vi "copy-data-eventSD.vi"(1 "cluster in":T1={"Kinetics"=[], "Spectrum"=[], "Experiments groups"=[], "GRAPH EXPERIMENTAL DATA"=[], "error out"={"status"=FALSE, "code"=0, "source"=""}, "group"=0, "exp selected"=0, "# exp"=0, "kinetics plot names"=[], "spectra plot names"=[], "FromToWave"={"FromWave"=0.0, "ToWave"=0.0}, "Laser shutter task"="", "Accelerator task"="", "Motor task"="", "GRAPH EXPERIMENTAL DATA ref"=refnum, "timedelays"=[0.0, 0.0, 0.0, 0.0, 0.0, 0.0, 0.0, 0.06019061100911815, 0.0521779104562645, 0.045231877429679615, 0.03921051490799832, 0.033990728811568754, 0.029465811603150715, 0.025543260876973825, 0.02214288834180205, 0.01919518054014414, 0.016639877791965713, 0.014424742312398925, 0.012504490320209958, 0.010839866306230088, 0.009396840537117498, 0.008145913389103785, 0.00706151229029317, 0.006121468943269439, 0.005306566140927374, 0.004600144911132549, 0.003987763959109073, 0.0034569044455719407, 0.00299671406541447, 0.0025977851951783253, 0.0022519625739982996, 0.00195217658646366, 0.0016922987392150965, 0.0014670163768006634, 0.0012717240756200802, 0.0011024294957352762, 0.0009556717658856477, 0.0008284507332614981, 0.0007181656316962257, 0.0006225619144775864, 0.0005396851648867825, 0.00046784114226338394, 0.0004055611468220084, 0.0003515719951773376, 0.00030476999279031153, 0.00026419837125694315, 0.00022902772919263772, 0.0001985390768670671, 0.0001721091379728629, 0.00014919760805372974, 0.00012933610911736794], "wavelengths"=[0.0, 0.0, 0.0, 0.0, 0.0, 0.0, 0.0, 0.06019061100911815, 0.0521779104562645, 0.045231877429679615, 0.03921051490799832, 0.033990728811568754, 0.029465811603150715, 0.025543260876973825, 0.02214288834180205, 0.01919518054014414, 0.016639877791965713, 0.014424742312398925, 0.012504490320209958, 0.010839866306230088, 0.009396840537117498, 0.008145913389103785, 0.00706151229029317, 0.006121468943269439, 0.005306566140927374, 0.004600144911132549, 0.003987763959109073, 0.0034569044455719407, 0.00299671406541447, 0.0025977851951783253, 0.0022519625739982996, 0.00195217658646366, 0.0016922987392150965, 0.0014670163768006634, 0.0012717240756200802, 0.0011024294957352762, 0.0009556717658856477, 0.0008284507332614981, 0.0007181656316962257, 0.0006225619144775864, 0.0005396851648867825, 0.00046784114226338394, 0.0004055611468220084, 0.0003515719951773376, 0.00030476999279031153, 0.00026419837125694315, 0.00022902772919263772, 0.0001985390768670671, 0.0001721091379728629, 0.00014919760805372974, 0.00012933610911736794], "Experiment"=refnum, "Commentaires exp"=refnum, "FromToDelay"={"FromDelay"=0.0, "ToDelay"=0.0}}, 2 "selected wavelengths":dbl[](array[numeric])=[550.0, 640.0, 680.0, 720.0, 780.0, 800.0], 3 "ItemTag":string) -> (0 "cluster out":T1={"Kinetics"=[], "Spectrum"=[], "Experiments groups"=[], "GRAPH EXPERIMENTAL DATA"=[], "error out"={"status"=FALSE, "code"=0, "source"=""}, "group"=0, "exp selected"=0, "# exp"=0, "kinetics plot names"=[], "spectra plot names"=[], "FromToWave"={"FromWave"=0.0, "ToWave"=0.0}, "Laser shutter task"="", "Accelerator task"="", "Motor task"="", "GRAPH EXPERIMENTAL DATA ref"=refnum, "timedelays"=[0.0, 0.0, 0.0, 0.0, 0.0, 0.0, 0.0, 0.06019061100911815, 0.0521779104562645, 0.045231877429679615, 0.03921051490799832, 0.033990728811568754, 0.029465811603150715, 0.025543260876973825, 0.02214288834180205, 0.01919518054014414, 0.016639877791965713, 0.014424742312398925, 0.012504490320209958, 0.010839866306230088, 0.009396840537117498, 0.008145913389103785, 0.00706151229029317, 0.006121468943269439, 0.005306566140927374, 0.004600144911132549, 0.003987763959109073, 0.0034569044455719407, 0.00299671406541447, 0.0025977851951783253, 0.0022519625739982996, 0.00195217658646366, 0.0016922987392150965, 0.0014670163768006634, 0.0012717240756200802, 0.0011024294957352762, 0.0009556717658856477, 0.0008284507332614981, 0.0007181656316962257, 0.0006225619144775864, 0.0005396851648867825, 0.00046784114226338394, 0.0004055611468220084, 0.0003515719951773376, 0.00030476999279031153, 0.00026419837125694315, 0.00022902772919263772, 0.0001985390768670671, 0.0001721091379728629, 0.00014919760805372974, 0.00012933610911736794], "wavelengths"=[0.0, 0.0, 0.0, 0.0, 0.0, 0.0, 0.0, 0.06019061100911815, 0.0521779104562645, 0.045231877429679615, 0.03921051490799832, 0.033990728811568754, 0.029465811603150715, 0.025543260876973825, 0.02214288834180205, 0.01919518054014414, 0.016639877791965713, 0.014424742312398925, 0.012504490320209958, 0.010839866306230088, 0.009396840537117498, 0.008145913389103785, 0.00706151229029317, 0.006121468943269439, 0.005306566140927374, 0.004600144911132549, 0.003987763959109073, 0.0034569044455719407, 0.00299671406541447, 0.0025977851951783253, 0.0022519625739982996, 0.00195217658646366, 0.0016922987392150965, 0.0014670163768006634, 0.0012717240756200802, 0.0011024294957352762, 0.0009556717658856477, 0.0008284507332614981, 0.0007181656316962257, 0.0006225619144775864, 0.0005396851648867825, 0.00046784114226338394, 0.0004055611468220084, 0.0003515719951773376, 0.00030476999279031153, 0.00026419837125694315, 0.00022902772919263772, 0.0001985390768670671, 0.0001721091379728629, 0.00014919760805372974, 0.00012933610911736794], "Experiment"=refnum, "Commentaires exp"=refnum, "FromToDelay"={"FromDelay"=0.0, "ToDelay"=0.0}})   [LabVIEW 2015]
uses:
  controls/control-cluster.ctl
  Classes/Experiments_group.lvclass
  globalVarSD.vi
  Classes/Experiment.lvclass
types:
  T1 = typedef "control-cluster.ctl" = cluster{"Kinetics":cluster{"timedelay":dbl[], dbl[]}[], "Spectrum":cluster{"Unités abscisse":dbl[], dbl[]}[], "Experiments groups":refnum<class "Experiments_group.lvclass">[], "GRAPH EXPERIMENTAL DATA":dbl[][], "error out":errorcluster, "group":i32, "exp selected":i32, "# exp":i32, "kinetics plot names":string[], "spectra plot names":string[], "FromToWave":cluster{"FromWave":dbl, "ToWave":dbl}, "Laser shutter task":refnum<k21>, "Accelerator task":refnum<k21>, "Motor task":refnum<k21>, "GRAPH EXPERIMENTAL DATA ref":refnum<vi>, "timedelays":dbl[], "wavelengths":dbl[], "Experiment":refnum<vi>, "Commentaires exp":refnum<vi>, "FromToDelay":cluster{"FromDelay":dbl, "ToDelay":dbl}}
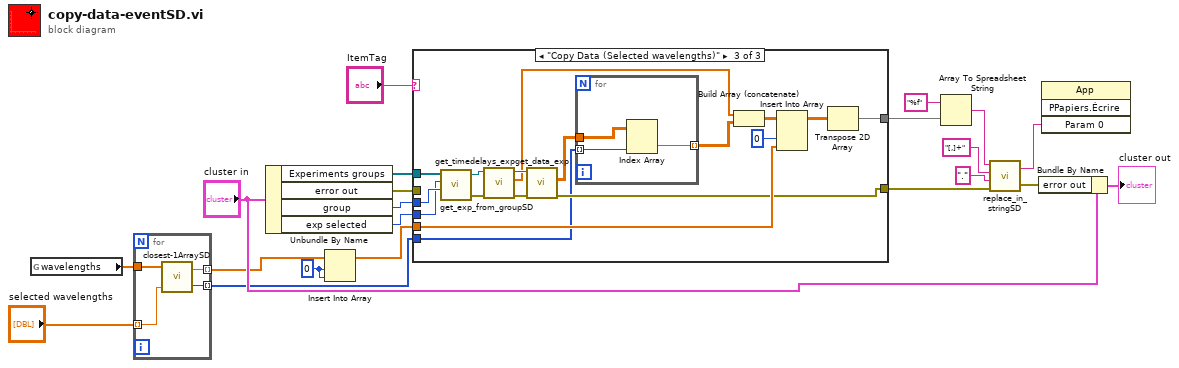
[diagram p0: block diagram]
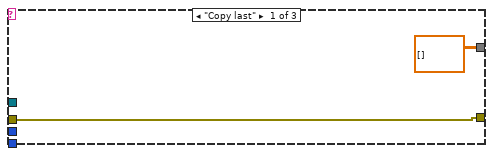
[diagram p2: hidden frame]
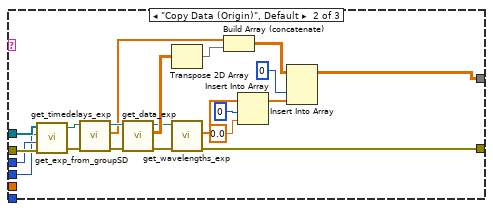
[diagram p3: hidden frame]
diagram:
  w2 = 0 ("index")
  n1 = global read "globalVarSD.vi" "wavelengths"() -> (w5:dbl[])
  n2 = for {
    tunnel: "selected wavelengths" -> [w24] mode=indexing
    tunnel: w5 -> [w25]
    tunnel: [w23] -> w1 mode=indexing
    tunnel: [w22] -> w4 mode=indexing
    n3 = call "closest-1ArraySD.vi"("desired element"=w24, "1D Array"=w25) -> ("closest index"=w23:i32, "closest element"=w22:dbl)  [unwired: 1 in]
  }
  n4 = Unbundle By Name("cluster in") -> ("Experiments groups"=w20:refnum<class "Experiments_group.lvclass">[], "error out"=w19:errorcluster, "group"=w15:i32, "exp selected"=w16:i32)
  n5 = Insert Into Array(array=w4, index=w2, new element=w2) -> (w3:dbl[])
  n6 = case shown="\"Copy Data (Selected wavelengths)\"" "ItemTag" {
    tunnel: [dbl[][] [] w36 w49] -> w17
    tunnel: [w26 w32 w54] -> w8
    tunnel: w20 -> [_ w31 w58]
    tunnel: w19 -> [w26 w30 _]
    tunnel: w15 -> [_ w29 w57]
    tunnel: w16 -> [_ w28 w56]
    tunnel: w3 -> [_ _ w55]
    tunnel: w1 -> [_ _ w53]
    frame "Copy last" {
    }
    frame "Copy Data (Origin)", Default {
      n7 = call "get_exp_from_groupSD.vi"("error in (no error)"=w30, "group"=w29, "exp selected"=w28, "Experiments groups"=w31) -> ("error out"=w35:errorcluster, "Experiment out"=w48:refnum<class "Experiment.lvclass">)  [unwired: 1 out]
      n8 = call-dynamic "get_timedelays_exp.vi"("error in (no error)"=w35, "Experiment.lvclass in"=w48) -> ("error out"=w34:errorcluster, "timedelays"=w46:dbl[], "Experiment.lvclass out"=w47:refnum<class "Experiment.lvclass">)  [unwired: 7 in]
      n9 = call-dynamic "get_data_exp.vi"("error in (no error)"=w34, "Experiment.lvclass in"=w47) -> ("error out"=w33:errorcluster, "Data"=w45:dbl[][], "Experiment.lvclass out"=w43:refnum<class "Experiment.lvclass">)  [unwired: 7 in]
      n10 = Transpose 2D Array(2D array=w45) -> (transposed array=w44:dbl[][])
      n11 = call-dynamic "get_wavelengths_exp.vi"("error in (no error)"=w33, "Experiment.lvclass in"=w43) -> ("error out"=w32:errorcluster, "wavelengths"=w42:dbl[])  [unwired: 7 in, 1 out]
      n12 = Build Array (concatenate)(w46, w44) -> (w39:dbl[][])
      n13 = Insert Into Array(array=w42, index=0, new element=0.0 ("new element/subarray")) -> (w37:dbl[])
      n14 = Insert Into Array(array=w39, index (col)=0 ("disabled index (col)"), new element=w37) -> (w36:dbl[][])  [unwired: 1 in]
    }
    frame "Copy Data (Selected wavelengths)" {
      n15 = call "get_exp_from_groupSD.vi"("group"=w57, "exp selected"=w56, "Experiments groups"=w58) -> ("error out"=w60:errorcluster, "Experiment out"=w65:refnum<class "Experiment.lvclass">)  [unwired: 1 in, 1 out]
      n16 = call-dynamic "get_timedelays_exp.vi"("error in (no error)"=w60, "Experiment.lvclass in"=w65) -> ("error out"=w59:errorcluster, "timedelays"=w63:dbl[], "Experiment.lvclass out"=w64:refnum<class "Experiment.lvclass">)  [unwired: 7 in]
      n17 = call-dynamic "get_data_exp.vi"("error in (no error)"=w59, "Experiment.lvclass in"=w64) -> ("error out"=w54:errorcluster, "Data"=w52:dbl[][])  [unwired: 7 in, 1 out]
      n18 = for {
        tunnel: w52 -> [w68]
        tunnel: w53 -> [w66] mode=indexing
        tunnel: [w67] -> w51 mode=indexing
        n19 = Index Array(array=w68, index (col)=w66) -> (element=w67:dbl[])  [unwired: 1 in]
      }
      n20 = Build Array (concatenate)(w63, w51) -> (w62:dbl[][])
      n21 = Insert Into Array(array=w62, index (col)=0 ("disabled index (col)"), new element=w55) -> (w50:dbl[][])  [unwired: 1 in]
      n22 = Transpose 2D Array(2D array=w50) -> (transposed array=w49:dbl[][])
    }
  }
  n23 = Array To Spreadsheet String(array=w17, 3:"%f" ("format string")) -> (spreadsheet string=w10:string)  [unwired: 1 in]
  n24 = call "replace_in_stringSD.vi"("error in (no error)"=w8, "replaced to.."=".", "characters to replace"="[,]+", "input string"=w10) -> ("error out"=w7:errorcluster, "output string"=w9:string)
  n25 = Bundle By Name(cluster="cluster in", "error out"=w7) -> (→"cluster out":T1)
  n26 = invoke class="App" method="PPapiers.Écrire"("Param 0"=w9) -> ()  [unwired: 3 in, 4 out]
